vi "pp2_cam_initalize.vi"(8 "error in":errorcluster, 11 "Camera":T2="cam0") -> (0 "error out":errorcluster, 2 "Image memory":T1, 3 "Session Out":T2)   [LabVIEW 2013]
uses:
  <vilib>/userdefined/High Color/IMAQdx.ctl
  <vilib>/vision/Image Controls.llb/IMAQ Image.ctl
  <vilib>/vision/driver/NI_Vision_Acquisition_Software.lvlib
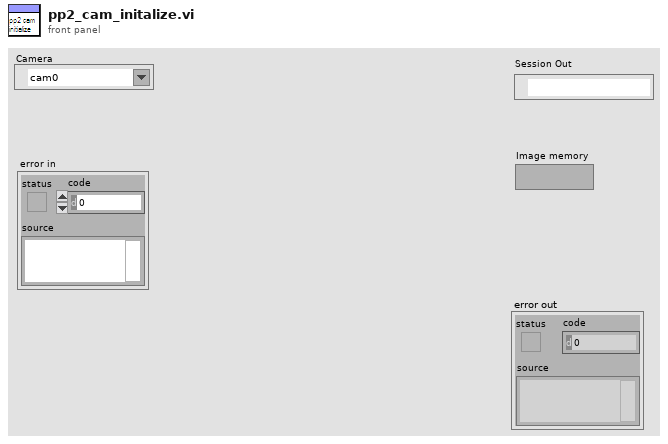
[diagram p1: front panel]
types:
  T1 = typedef "IMAQ Image.ctl" = refnum<image>
  T2 = typedef "IMAQdx.ctl" = refnum<k21>
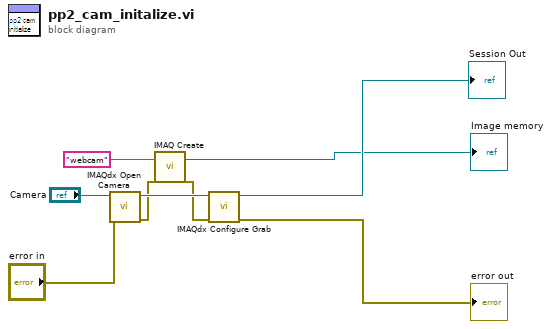
[diagram p0: block diagram]
diagram:
  n1 = call <vilib>:"IMAQdx Open Camera.vi"("error in"="error in", "Session In"="Camera") -> ("error out"=w6:errorcluster, "Session Out"=w9:T2)  [unwired: 8 in]
  n2 = call "IMAQ Create"("Image Name"="webcam", "error in (no error)"=w6) -> ("New Image"=→"Image memory":T1, "error out"=w5:errorcluster)  [unwired: 3 in]
  n3 = call <vilib>:"IMAQdx Configure Grab.vi"("error in"=w5, "Session In"=w9) -> ("error out"=→"error out":errorcluster, "Session Out"=→"Session Out":T2)  [unwired: 8 in]
